vi "Live camera test.vi"(8 "Gain":i32 min=100 max=2000 step=1, 9 "Exposure time (ms)":dbl=100.0 min=1.0 max=10000.0 step=1.0) -> (2 "Image out":T1(plugin-control))   [LabVIEW 2017]
panel:
  in  "stop":bool
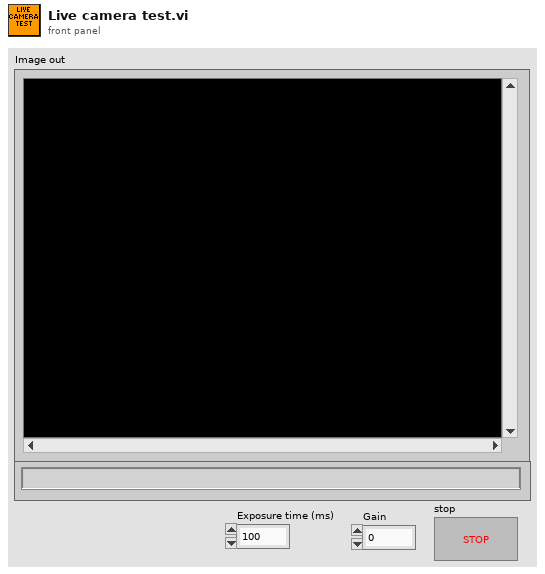
[diagram p1: front panel]
types:
  T1 = typedef "IMAQ Image.ctl" = refnum<image>
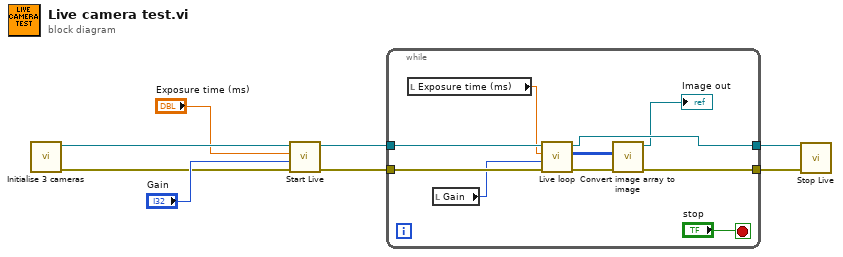
[diagram p0: block diagram]
diagram:
  n1 = call "Initialise 3 cameras.vi"() -> ("Error Out"=w5:errorcluster, "Red camera ref"=w8:refnum<k24>)  [unwired: 8 in, 2 out]
  n2 = call "Start Live.vi"("Error In"=w5, "Gain in"="Gain", "Exposure time (ms)"="Exposure time (ms)", "Camera reference in"=w8) -> ("Error Out"=w1:errorcluster, "Camera reference out"=w2:refnum<k24>)  [unwired: 5 in]
  n3 = while {
    tunnel: [w10] -> w4
    tunnel: [w17] -> w3
    tunnel: w2 -> [w16]
    tunnel: w1 -> [w15]
    stop <- "stop" stop-if-true
    n4 = local read "Exposure time (ms)"() -> (w14:dbl)
    n5 = local read "Gain"() -> (w13:i32)
    n6 = call "Live loop.vi"("Error In"=w15, "Gain"=w13, "Exposure time (ms)"=w14, "Camera reference in"=w16) -> ("Error Out"=w11:errorcluster, "Image Array"=w12:u16[][], "Camera reference out"=w17:refnum<k24>)  [unwired: 4 in]
    n7 = call "Convert image array to image.vi"("Error In"=w11, "Array"=w12) -> ("error out"=w10:errorcluster, "Image Out"=→"Image out":T1)  [unwired: 7 in]
  }
  n8 = call "Stop Live.vi"("Camera reference in"=w3, "Error In"=w4) -> ()  [unwired: 16 in, 2 out]
